vi "_iv_AUTO3.vi"(5 "i-v class":T1={"start(mV)"=0.0, "stop(mV)"=5.0, "step(mV)"=0.1, "file_name"="IV-TRx_0.00_111_test.csv", "IF OFF/ON"=TRUE, "SAVE OFF/ON"=TRUE, "frq(GHz)"=8.0, "avg"=1, "Sweep mode"=1, "VminfromSS"=0.05, "Measurement mode"=1, "Vopt"=0} {"Measurement mode" items=["Voltage sweep", "Every time HOT/COLD"]; "Sweep mode" items=["Once", "Hot/Cold auto", "HOT/Cold Manula"]}, 6 "Control":T3={"GPIB_ATT"="28", "6501Dev#"=1, "GPIB_SP"="18", "GPIB_PM"="13", "GPIB_DSA"="11", "GPIB_DMM (TPD)"="23", "GPIB_MPI"="2", "mortor setup"=[{"Axis"=0, "ID"=0, "HIspeed"=200.0, "LOspeed"=100.0, "ACCEL(ms)"=100.0, "Sratio"=50.0, "free ride"=TRUE, "string"="DSB HOT/COLD"}, {"Axis"=1, "ID"=0, "HIspeed"=4.0, "LOspeed"=4.0, "ACCEL(ms)"=100.0, "Sratio"=50.0, "free ride"=TRUE, "string"="SubMM Att"}], "DATA path"=path "Z:/band10/Labview_ALMA/MIX95/test", "DB path"=path "Z:/band10/Labview_ALMA/MIX95/test", "comment"="P1_Tmin", "ColdCarts"="003601", "Th"=295.0, "Tc"=77.0, "Set_SIS_volt"=2.1, "Offset"=0.0, "control"=0, "FreqLO"=800.0, "Set_Mag_Cur"=800.0, "MPI offset(mm)"=22.99, "HOT/COLD"=0} {"HOT/COLD" items=["DSB", "SBR", "GainComp"]; "control" items=["CLOSE LOOP", "OPEN LOOP", "Not Control"]}, 7 "Bias_LO_equip":T2={"Node address"=19, "CAN Interface"="CAN0", "Cartridge band"=10, "Slave Node in"={"Address"=0, "Serial Number"=[]}, "ObjHandle out"=0, "POL"=1, "sb"=1, "GPIB_SM (SIS S,V)"="24", "GPIB_DMM (SIS I)"="22", "GPIB_SM (MAG I) "="25", "GPIB_SG(LO)"="19", "GPIB_PW (PAMP) "="6", "GPIB_TMP1(8ch)"="12", "GPIB_TMP2(2ch)  "="13", "WCA_avg"=10, "Rsen"=10.0, "BiasModule"=1, "LOModule "=1, "WCA_LO_FREQ_SET"={"YTO Low freq. [GHz]"=14.42, "YTO High freq. [GHz]"=17.7, "Kvco"=1, "Lock Pol."=0, "SET LO FREQ"=72.5, "Multiplier"=6.0, "YTO (HEX)"=0, "YTO coarse( FREQ)"=25.0, "NULL PLL INTEGRATOR"=FALSE}, "Res for"=0} {"Res for" items=["none", "series res", "parallel res"]; "WCA_LO_FREQ_SET"."YTO coarse( FREQ)" min=25 max=150 step=0.0001 format="%.3f"; "WCA_LO_FREQ_SET"."Multiplier" min=3 max=6 step=3; "WCA_LO_FREQ_SET"."SET LO FREQ" min=25 max=150 step=0.0001 format="%.3f"; "WCA_LO_FREQ_SET"."Lock Pol." items=["Lower", "Upper"]; "WCA_LO_FREQ_SET"."Kvco" items=["7.5MHz/V", "15MHz/V"]; "WCA_LO_FREQ_SET"."YTO High freq. [GHz]" format="%.3f"; "WCA_LO_FREQ_SET"."YTO Low freq. [GHz]" format="%.3f"; "LOModule" items=["Manual", "B10Lab LO", "WCA LO"]; "BiasModule" items=["B10Lab Bias", "WCA BiasModule"]; "Slave Node in"."Serial Number" format="%.0x"; "Slave Node in"."Address" format="%.0x"; "Cartridge band" max=10 step=1; "Node address" format="%.0x"}) -> (0 "Output string":string, 1 "Set_SIS_volt":dbl=2.1, 2 "XY graph 3":cluster{dbl[], dbl[]}(graph), 3 "XY graph 2":cluster{dbl[], dbl[]}(graph))   [LabVIEW 2017]
uses:
  Instance           3 17Saved   _iv_AUTO3 .vi
  Instance           2 17Saved   _iv_AUTO3 .vi
  <vilib>/express/express shared/transition.llb/Dynamic To Waveform Array.vi
  <vilib>/express/express arith-compare/Formula/Block/exnFormulaBlock how many pts in the wave.vi
  <vilib>/express/express shared/ex_Modify Signal Name.vi
  <vilib>/express/express shared/transition.llb/Waveform Array To Dynamic.vi
  Instance           4 17Saved   _iv_AUTO3 .vi
  <vilib>/express/express arith-compare/Formula/XNode/ExpressFormulaBlockNode.xnode
panel:
  in  "Controller":enum32{"Page 1", "Page 2"}(tab)=enum."Page 2"
  out "XY graph":cluster{dbl[], dbl[]}[](graph)
  out "string":string
  in  "OK":bool
  # "LO freq. [GHz]"
  # "YTO LOW\n/High Freq."
  # "ZERO Intgrtr"
  # "Node Address"
  # "Serial Number"
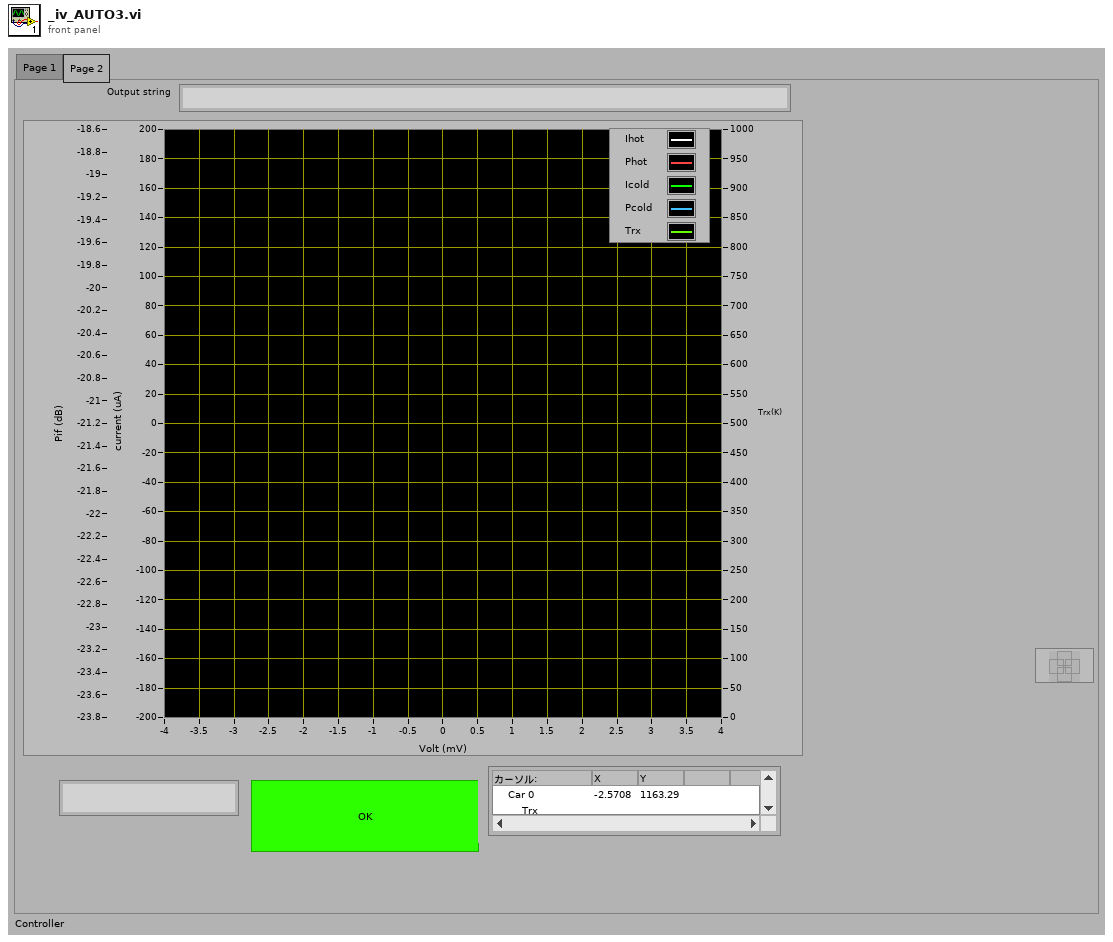
[diagram p1: front panel]
types:
  T1 = cluster{"start(mV)":dbl, "stop(mV)":dbl, "step(mV)":dbl, "file_name":string, "IF OFF/ON":bool, "SAVE OFF/ON":bool, "frq(GHz)":dbl, "avg":i32, "Sweep mode":u16, "VminfromSS":dbl, "Measurement mode":u16, "Vopt":u16}
  T2 = cluster{"Node address":u16, "CAN Interface":string, "Cartridge band":u32, "Slave Node in":cluster{"Address":i16, "Serial Number":i8[]}, "ObjHandle out":u32, "POL":u32, "sb":u32, "GPIB_SM (SIS S,V)":string, "GPIB_DMM (SIS I)":string, "GPIB_SM (MAG I) ":string, "GPIB_SG(LO)":string, "GPIB_PW (PAMP) ":string, "GPIB_TMP1(8ch)":string, "GPIB_TMP2(2ch)  ":string, "WCA_avg":i32, "Rsen":dbl, "BiasModule":u16, "LOModule ":u16, "WCA_LO_FREQ_SET":cluster{"YTO Low freq. [GHz]":sgl, "YTO High freq. [GHz]":sgl, "Kvco":u16, "Lock Pol.":u16, "SET LO FREQ":sgl, "Multiplier":sgl, "YTO (HEX)":u16, "YTO coarse( FREQ)":sgl, "NULL PLL INTEGRATOR":bool}, "Res for":u16}
  T3 = cluster{"GPIB_ATT":string, "6501Dev#":i16, "GPIB_SP":string, "GPIB_PM":string, "GPIB_DSA":string, "GPIB_DMM (TPD)":string, "GPIB_MPI":string, "mortor setup":cluster{"Axis":i16, "ID":i16, "HIspeed":dbl, "LOspeed":dbl, "ACCEL(ms)":dbl, "Sratio":dbl, "free ride":bool, "string":string}[], "DATA path":path, "DB path":path, "comment":string, "ColdCarts":string, "Th":dbl, "Tc":dbl, "Set_SIS_volt":dbl, "Offset":dbl, "control":u16, "FreqLO":dbl, "Set_Mag_Cur":dbl, "MPI offset(mm)":dbl, "HOT/COLD":u16}
  T4 = cluster{"Axis":i16, "ID":i16, "HIspeed":dbl, "LOspeed":dbl, "ACCEL(ms)":dbl, "Sratio":dbl, "free ride":bool, "string":string}[]
  T5 = cluster{"Axis":i16, "ID":i16, "HIspeed":dbl, "LOspeed":dbl, "ACCEL(ms)":dbl, "Sratio":dbl, "free ride":bool, "string":string}
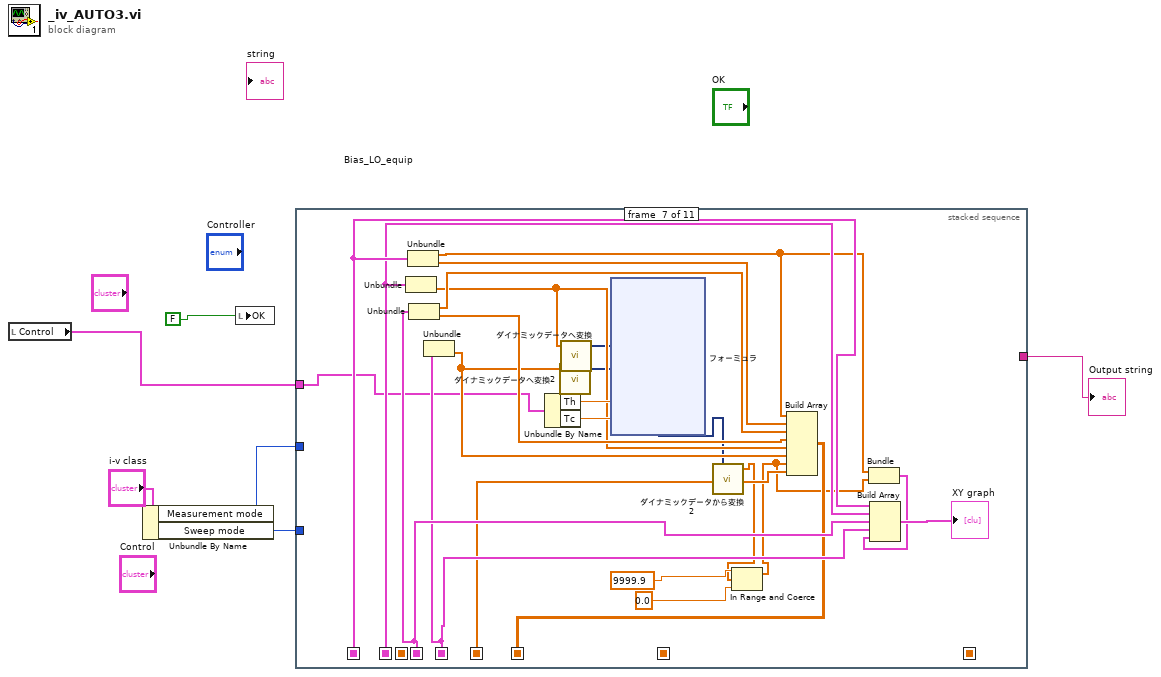
[diagram p0: block diagram]
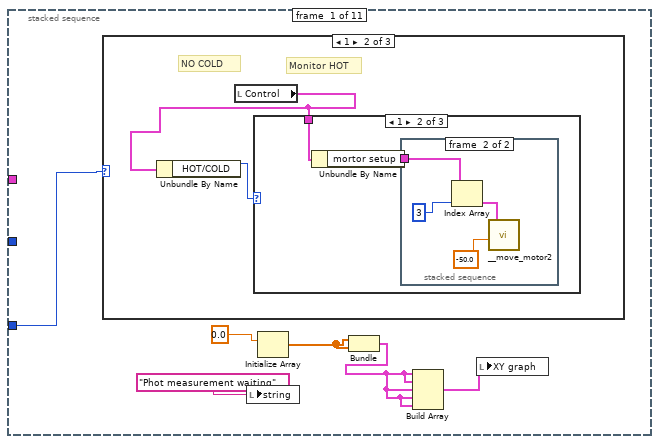
[diagram p2: hidden frame]
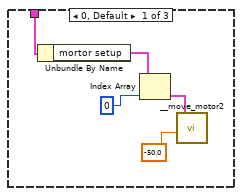
[diagram p4: hidden frame]
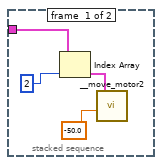
[diagram p5: hidden frame]
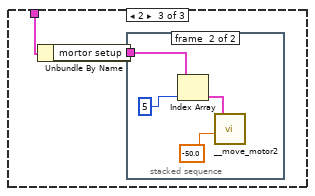
[diagram p6: hidden frame]
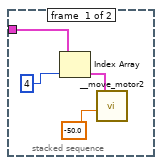
[diagram p7: hidden frame]
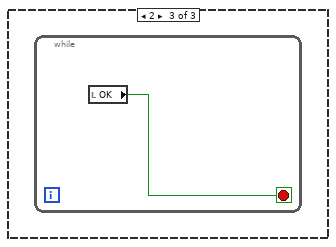
[diagram p8: hidden frame]
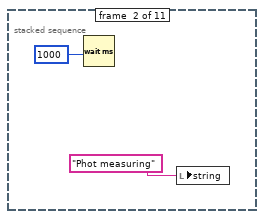
[diagram p9: hidden frame]
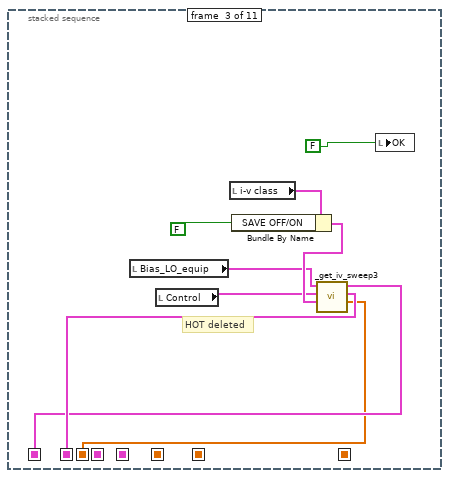
[diagram p10: hidden frame]
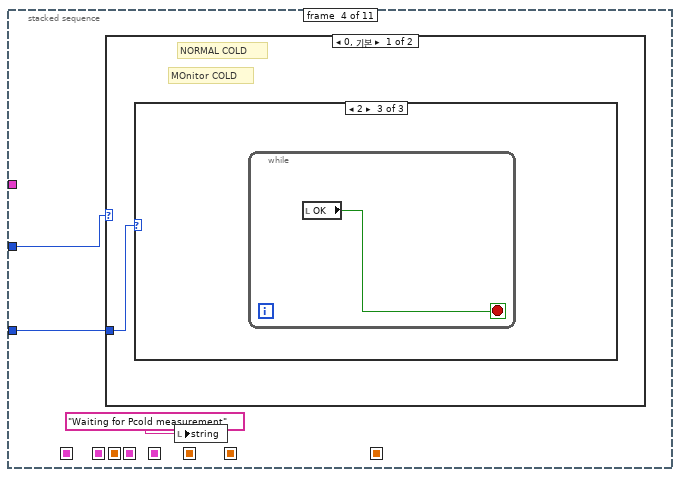
[diagram p11: hidden frame]
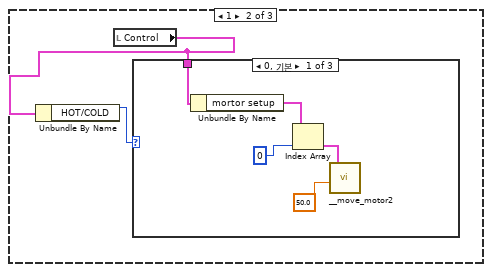
[diagram p13: hidden frame]
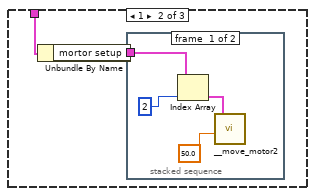
[diagram p14: hidden frame]
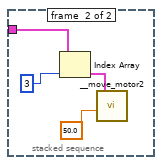
[diagram p15: hidden frame]
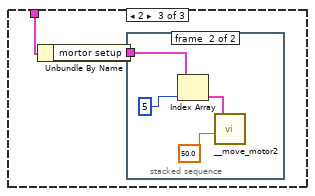
[diagram p16: hidden frame]
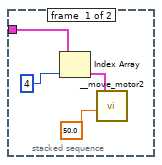
[diagram p17: hidden frame]
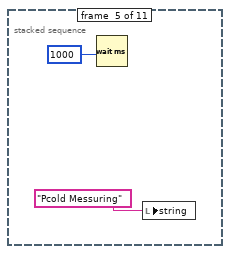
[diagram p19: hidden frame]
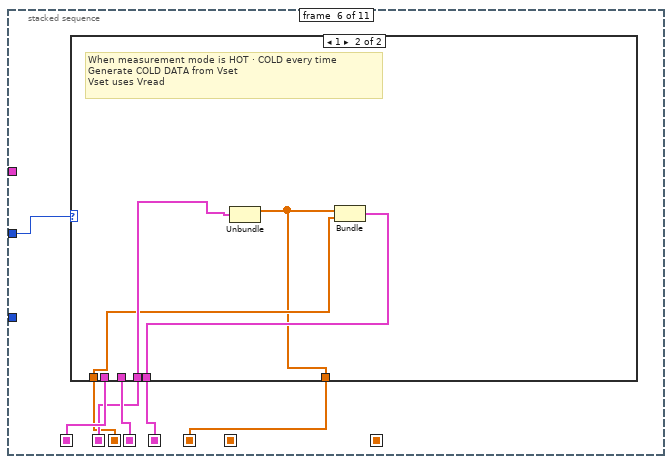
[diagram p20: hidden frame]
diagram:
  n1 = local read "Control"() -> (w5:T3)
  n2 = Unbundle By Name("i-v class") -> ("Measurement mode"=w3:u16, "Sweep mode"=w2:u16)
  n3 = local write "OK"(FALSE) -> ()
  n4 = stacked-sequence {
    seq-local: [_ _ w45 _ _ _ _ _ _ _ _] -> [_ _ _ _ _ w88 w125 _ _ _ _]
    seq-local: [_ _ w50 _ _ _ _ _ _ _ _] -> [_ _ _ _ _ w87 w124 _ _ _ _]
    seq-local: [_ _ _ _ _ w91 _ _ _ _ _] -> [_ _ _ _ _ _ w123 _ _ _ _]
    seq-local: [_ _ _ _ _ w90 _ _ _ _ _] -> [_ _ _ _ _ _ w122 _ _ _ _]
    seq-local: [_ _ _ _ _ w92 _ _ _ _ _] -> [_ _ _ _ _ _ w112 _ _ _ _]
    seq-local: [_ _ _ _ _ _ w110 _ _ _ _] -> [_ _ _ _ _ _ _ w271 w289 _ _]
    seq-local: [_ _ _ _ _ _ _ _ w290 _ _] -> [_ _ _ _ _ _ _ _ _ w356 _]
    seq-local: [_ _ _ _ _ _ _ _ _ w339 _] -> [_ _ _ _ _ _ _ _ _ _ w372]
    seq-local: [_ _ w44 _ _ _ _ _ _ _ _] -> [_ _ _ _ _ w86 _ _ _ _ _]
    tunnel: w5 -> [_ _ _ _ _ _ w109 w268 _ _ _]
    tunnel: [_ _ _ _ _ _ _ _ _ w338 _] -> w6
    tunnel: w3 -> [_ _ _ w54 _ w89 _ _ _ _ _]
    tunnel: w2 -> [w8 _ _ w53 _ _ _ _ _ _ _]
    frame #0 {
      n5 = case shown="1" w8 {
        frame 0, Default {
        }
        frame 1 {
          # "NO COLD"
          # "Monitor HOT"
          n6 = local read "Control"() -> (w13:T3)
          n7 = Unbundle By Name(w13) -> ("HOT/COLD"=w14:u16)
          n8 = case shown="1" w14 {
            tunnel: w13 -> [w17 w21 w31]
            frame 0, Default {
              n9 = Unbundle By Name(w17) -> ("mortor setup"=w16:T4)
              n10 = Index Array(array=w16, index=0) -> (element=w15:T5)
              n11 = call "__move_motor2.vi"("Moving distance"=-50.0, "motor setup"=w15) -> ()  [unwired: 2 in, 2 out]
            }
            frame 1 {
              n12 = Unbundle By Name(w21) -> ("mortor setup"=w20:T4)
              n13 = stacked-sequence {
                tunnel: w20 -> [w23 w27]
                frame #0 {
                  n14 = Index Array(array=w23, index=2) -> (element=w22:T5)
                  n15 = call "__move_motor2.vi"("Moving distance"=-50.0, "motor setup"=w22) -> ()  [unwired: 2 in, 2 out]
                }
                frame #1 {
                  n16 = Index Array(array=w27, index=3) -> (element=w26:T5)
                  n17 = call "__move_motor2.vi"("Moving distance"=-50.0, "motor setup"=w26) -> ()  [unwired: 2 in, 2 out]
                }
              }
            }
            frame 2 {
              n18 = Unbundle By Name(w31) -> ("mortor setup"=w30:T4)
              n19 = stacked-sequence {
                tunnel: w30 -> [w33 w37]
                frame #0 {
                  n20 = Index Array(array=w33, index=4) -> (element=w32:T5)
                  n21 = call "__move_motor2.vi"("Moving distance"=-50.0, "motor setup"=w32) -> ()  [unwired: 2 in, 2 out]
                }
                frame #1 {
                  n22 = Index Array(array=w37, index=5) -> (element=w36:T5)
                  n23 = call "__move_motor2.vi"("Moving distance"=-50.0, "motor setup"=w36) -> ()  [unwired: 2 in, 2 out]
                }
              }
            }
          }
        }
        frame 2 {
          n24 = while {
            stop <- w40 stop-if-true
            n25 = local read "OK"() -> (w40:bool)
          }
        }
      }
      n26 = local write "string"("Phot measurement waiting") -> ()
      n27 = Initialize Array(0.0) -> (w12:dbl[])  [unwired: 1 in]
      n28 = Bundle(w12, w12) -> (w9:cluster{dbl[], dbl[]})  [unwired: 1 in]
      n29 = Build Array(w9, w9, w9, w9, w9) -> (w10:cluster{dbl[], dbl[]}[])
      n30 = local write "XY graph"(w10) -> ()
    }
    frame #1 {
      n31 = Wait (ms)(milliseconds to wait=1000) -> ()  [unwired: 1 out]
      n32 = local write "string"("Phot measuring") -> ()
    }
    frame #2 {
      # "HOT deleted"
      n33 = local read "Bias_LO_equip"() -> (w47:T2)
      n34 = local read "Control"() -> (w46:T3)
      n35 = local read "i-v class"() -> (w49:T1)
      n36 = Bundle By Name(cluster=w49, "SAVE OFF/ON"=FALSE) -> (w48:T1)
      n37 = call "_get_iv_sweep3.vi"("I-V class"=w48, "Control"=w46, "Bias_LO_equip"=w47) -> ("Vset"=w44:dbl[], "VP class"=w50:cluster{"array":dbl[], "array2":dbl[]}, "VI class"=w45:cluster{"array":dbl[], "array2":dbl[]})  [unwired: 2 in]
      n38 = local write "OK"(FALSE) -> ()
    }
    frame #3 {
      n39 = case shown="0, 기본" w54 {
        tunnel: w53 -> [w55 _]
        frame 0, Default {
          # "NORMAL COLD"
          # "MOnitor COLD"
          n40 = case shown="2" w55 {
            frame 0, Default {
            }
            frame 1 {
              n41 = local read "Control"() -> (w56:T3)
              n42 = Unbundle By Name(w56) -> ("HOT/COLD"=w57:u16)
              n43 = case shown="0, 기본" w57 {
                tunnel: w56 -> [w60 w64 w74]
                frame 0, Default {
                  n44 = Unbundle By Name(w60) -> ("mortor setup"=w59:T4)
                  n45 = Index Array(array=w59, index=0) -> (element=w58:T5)
                  n46 = call "__move_motor2.vi"("Moving distance"=50.0, "motor setup"=w58) -> ()  [unwired: 2 in, 2 out]
                }
                frame 1 {
                  n47 = Unbundle By Name(w64) -> ("mortor setup"=w63:T4)
                  n48 = stacked-sequence {
                    tunnel: w63 -> [w66 w70]
                    frame #0 {
                      n49 = Index Array(array=w66, index=2) -> (element=w65:T5)
                      n50 = call "__move_motor2.vi"("Moving distance"=50.0, "motor setup"=w65) -> ()  [unwired: 2 in, 2 out]
                    }
                    frame #1 {
                      n51 = Index Array(array=w70, index=3) -> (element=w69:T5)
                      n52 = call "__move_motor2.vi"("Moving distance"=50.0, "motor setup"=w69) -> ()  [unwired: 2 in, 2 out]
                    }
                  }
                }
                frame 2 {
                  n53 = Unbundle By Name(w74) -> ("mortor setup"=w73:T4)
                  n54 = stacked-sequence {
                    tunnel: w73 -> [w77 w80]
                    frame #0 {
                      n55 = Index Array(array=w77, index=4) -> (element=w76:T5)
                      n56 = call "__move_motor2.vi"("Moving distance"=50.0, "motor setup"=w76) -> ()  [unwired: 2 in, 2 out]
                    }
                    frame #1 {
                      n57 = Index Array(array=w80, index=5) -> (element=w79:T5)
                      n58 = call "__move_motor2.vi"("Moving distance"=50.0, "motor setup"=w79) -> ()  [unwired: 2 in, 2 out]
                    }
                  }
                }
              }
            }
            frame 2 {
              n59 = while {
                stop <- w83 stop-if-true
                n60 = local read "OK"() -> (w83:bool)
              }
            }
          }
        }
        frame 1 {
          # "When the measurement mode is HOT / COLD every time, do nothing"
        }
      }
      n61 = local write "string"("Waiting for Pcold measurement") -> ()
    }
    frame #4 {
      n62 = Wait (ms)(milliseconds to wait=1000) -> ()  [unwired: 1 out]
      n63 = local write "string"("Pcold Messuring") -> ()
    }
    frame #5 {
      n64 = case shown="1" w89 {
        tunnel: [w96 w100] -> w92
        tunnel: [w94 w104] -> w91
        tunnel: [w93 w101] -> w90
        tunnel: w88 -> [_ w104]
        tunnel: w87 -> [_ w103]
        tunnel: w86 -> [_ w102]
        frame 0, Default {
          # "COLD data acquisition"
          n65 = local read "Bias_LO_equip"() -> (w95:T2)
          n66 = local read "i-v class"() -> (w98:T1)
          n67 = Bundle By Name(cluster=w98, "SAVE OFF/ON"=FALSE) -> (w97:T1)
          n68 = call "_get_iv_sweep3.vi"("I-V class"=w97, "Bias_LO_equip"=w95) -> ("Vset"=w96:dbl[], "VP class"=w93:cluster{"array":dbl[], "array2":dbl[]}, "VI class"=w94:cluster{"array":dbl[], "array2":dbl[]})  [unwired: 3 in]
          "XY graph 2" <- w94
          "XY graph 3" <- w93
        }
        frame 1 {
          # "When measurement mode is HOT · COLD every time\nGenerate COLD DATA from Vset\nVset uses Vread"
          n69 = Unbundle(w103) -> ("array"=w100:dbl[])  [unwired: 1 out]
          n70 = Bundle("array"=w100, "Vset"=w102) -> (w101:cluster{"array":dbl[], "Vset":dbl[]})  [unwired: 1 in]
        }
      }
    }
    frame #6 {
      n71 = Unbundle(w124) -> ("array2"=w117:dbl[])  [unwired: 1 out]
      n72 = Unbundle(w125) -> ("array"=w121:dbl[], "array2"=w127:dbl[])
      n73 = Unbundle(w123) -> ("array"=w126:dbl[], "array2"=w128:dbl[])
      n74 = Unbundle(w122) -> ("Vset"=w115:dbl[])  [unwired: 1 out]
      n75 = Unbundle By Name(w109) -> ("Th"=w119:dbl, "Tc"=w118:dbl)
      n76 = call "ダイナミックデータへ変換2"("Array"=w115) -> ("Dynamic Data Type"=w114:dynamicdata)  [unwired: 3 in]
      n77 = call "ダイナミックデータへ変換"("Array"=w117) -> ("Dynamic Data Type"=w116:dynamicdata)  [unwired: 3 in]
      n78 = xnode "フォーミュラ"("Ph"=w116, "Pc"=w114, "th"=w119, "tc"=w118) -> ("결과"=w113:dynamicdata)  [unwired: 1 in, 1 out]
      n79 = call "ダイナミックデータから変換2"("Dynamic Data Type"=w113) -> ("Array"=w106:dbl[])  [unwired: 3 in]
      n80 = In Range and Coerce(upper limit=9999.9, x=w106, lower limit=0.0) -> (coerced(x)=w105:dbl[])  [unwired: 1 out]
      n81 = Build Array(w121, w127, w126, w128, w117, w115, w105, w112) -> (w110:dbl[][])
      n82 = Bundle("array"=w121, w105) -> (w111:cluster{"array":dbl[], dbl[]})  [unwired: 1 in]
      n83 = Build Array(w125, w124, w123, w122, w111) -> (→"XY graph":cluster{"array":dbl[], "Vset":dbl[]}[])
    }
    frame #7 {
      n84 = local read "i-v class"() -> (w269:T1)
      n85 = Unbundle By Name(w269) -> ("SAVE OFF/ON"=w270:bool)
      n86 = case shown="참" w270 {
        tunnel: w271 -> [_ w278]
        tunnel: w269 -> [_ w276]
        tunnel: w268 -> [_ w274]
        frame False {
        }
        frame True {
          n87 = Unbundle By Name(w276) -> ("file_name"=w275:string)
          n88 = Unbundle By Name(w274) -> ("DATA path"=w273:path, "Offset"=w272:dbl)
          n89 = Format Into String(format string="Vsis,Ihot,Vcold,Icold,Phot,Pcold,Trx,Vset with Offset=%f", w272) -> (resulting string=w279:string)  [unwired: 2 in, 1 out]
          n90 = call "___save_2d_data_with_header.vi"("ヘッダー"=w279, "”z—ñ"=w278, "Œ`Ž®"="%^.3e", "file_name"=w275, "パス"=w273) -> ()  [unwired: 6 in, 1 out]
        }
      }
    }
    frame #8 {
      n91 = local read "i-v class"() -> (w285:T1)
      n92 = local read "Control"() -> (w287:T3)
      n93 = Unbundle By Name(w285) -> ("Vopt"=w281:u16, "VminfromSS"=w283:dbl)
      n94 = Array Size(array=w289) -> (size(s)=w293:i32[])
      n95 = Index Array(array=w293, index=1) -> (element=w291:i32)
      n96 = Unbundle By Name(w287) -> ("FreqLO"=w286:dbl)
      n97 = expression code="2.0678E -3*x"(w286) -> (w284:dbl)
      n98 = Add(x=w284, y=w283) -> (x+y=w282:dbl)
      n99 = case shown="1" w281 {
        tunnel: w291 -> [_ w299 w319]
        tunnel: [w294 w298 w318] -> w290
        tunnel: w289 -> [w294 w297 w317]
        tunnel: dbl[][] [] -> [_ w296 w316]
        tunnel: w282 -> [_ w295 w315]
        frame 0, Default {
        }
        frame 1 {
          n100 = for {
            N: w299 -> [_]
            tunnel: w297 -> [w306]
            shift-right: [w305] -> w298
            shift-left: w296 -> [w304]
            tunnel: w295 -> [w300]
            i -> [w302]
            n101 = Index Array(array=w306, index (row)=0, index (col)=w302) -> (element=w308:dbl)
            n102 = In Range and Coerce(upper limit=2.3, x=w308, lower limit=w300) -> (In Range?=w307:bool)  [unwired: 1 out]
            n103 = case shown="참" w307 {
              tunnel: w302 -> [_ w310]
              tunnel: w306 -> [_ w314]
              tunnel: [w309 w312] -> w305
              tunnel: w304 -> [w309 w311]
              frame False {
              }
              frame True {
                n104 = Index Array(array=w314, index (col)=w310) -> (element=w313:dbl[])  [unwired: 1 in]
                n105 = Build Array (concatenate)(w311, w313) -> (w312:dbl[][])
              }
            }
          }
        }
        frame 2 {
          n106 = for {
            N: w319 -> [_]
            tunnel: w317 -> [w327]
            shift-right: [w326] -> w318
            shift-left: w316 -> [w325]
            tunnel: w315 -> [w320]
            i -> [w323]
            n107 = Index Array(array=w327, index (row)=0, index (col)=w323) -> (element=w329:dbl)
            n108 = Negate(x=w320) -> (-x=w321:dbl)
            n109 = In Range and Coerce(upper limit=w321, x=w329, lower limit=-2.3) -> (In Range?=w328:bool)  [unwired: 1 out]
            n110 = case shown="참" w328 {
              tunnel: w323 -> [_ w331]
              tunnel: w327 -> [_ w335]
              tunnel: [w330 w333] -> w326
              tunnel: w325 -> [w330 w332]
              frame False {
              }
              frame True {
                n111 = Index Array(array=w335, index (col)=w331) -> (element=w334:dbl[])  [unwired: 1 in]
                n112 = Build Array (concatenate)(w332, w334) -> (w333:dbl[][])
              }
            }
          }
        }
      }
    }
    frame #9 {
      n113 = Index Array(array=w356, index (col)=6) -> (element=w358:dbl[])  [unwired: 1 in]
      n114 = Array Size(array=w358) -> (size(s)=w357:i32)
      n115 = for {
        N: w357 -> [_]
        tunnel: w358 -> [w367]
        tunnel: [w363] -> w359 mode=indexing
        i -> [w368]
        n116 = Index Array(array=w367, index=w368) -> (element=w362:dbl)
        n117 = In Range and Coerce(upper limit=9999.9, x=w362, lower limit=80.0) -> (In Range?=w364:bool)  [unwired: 1 out]
        n118 = case shown="참" w364 {
          tunnel: [9999.9 w370] -> w363
          tunnel: w362 -> [_ w370]
          frame False {
          }
          frame True {
          }
        }
      }
      n119 = Array Max & Min(array=w359) -> (min index (indices)=w360:i32)  [unwired: 3 out]
      n120 = Index Array(array=w356, index (row)=w360) -> (element=w361:dbl[])  [unwired: 1 in]
      n121 = Get Date/Time In Seconds() -> (seconds since 1Jan1904=w354:timestamp)
      n122 = Format Date/Time String(time format string (%c)="%Y-%m-%d  %H:%M:%S", seconds (now)=w354) -> (date/time string=w344:string)  [unwired: 1 in]
      n123 = local read "Control"() -> (w337:T3)
      n124 = local read "Bias_LO_equip"() -> (w355:T2)
      n125 = formula code="float32 VJ,IJ;\nfloat32 Vset,Trx,Ph,Pc;\nVJ=ar[0];\nIJ=ar[1];\nVset=ar[7];\nPh=ar[4];\nPc=ar[5];\nTrx=ar[6];"("ar"=w361) -> ("VJ"=w347:sgl, "IJ"=w346:sgl, "Trx"=w348:sgl, "Vset"=w339:sgl, "Ph"=w350:sgl, "Pc"=w349:sgl)
      n126 = Unbundle By Name(w337) -> ("FreqLO"=w351:dbl)
      n127 = Unbundle By Name(w337) -> ("comment"=w340:string)
      n128 = Unbundle By Name(w355) -> ("BiasModule"=w343:u16, "LOModule"=w342:u16, "POL"=w341:u32)
      n129 = Unbundle By Name(w337) -> ("Offset"=w345:dbl)
      n130 = Format Into String(format string="IVTrx,%.2f,%2.2f,%2.2f,%.1f,%2.2f,%4.1f,%2.2f,%.3f,%s,%d,%d,%d,%s", w351, w350, w349, w348, w347, w346, w339, w345, w344, w343, w342, w341, w340) -> (resulting string=w338:string)  [unwired: 2 in, 1 out]
    }
    frame #10 {
      n131 = local read "i-v class"() -> (w375:T1)
      n132 = Unbundle By Name(w375) -> ("Vopt"=w374:u16)
      n133 = case shown="0, 기본" w374 {
        tunnel: w372 -> [w376 _]
        tunnel: [w376 w381] -> w371
        frame 1, 2 {
          n134 = local read "Control"() -> (w377:T3)
          n135 = local read "Bias_LO_equip"() -> (w378:T2)
          n136 = Unbundle By Name(w377) -> ("Offset"=w380:dbl, "control"=w379:u16)
          n137 = call "__SISbias_Set.vi"("SIS@Mode"=w379, "Offset"=w380, "Set_V"=w376, "Bias_LO_equip"=w378) -> ()  [unwired: 7 in, 1 out]
        }
        frame 0, Default {
          n138 = local read "Control"() -> (w382:T3)
          n139 = local read "Bias_LO_equip"() -> (w383:T2)
          n140 = Unbundle By Name(w382) -> ("Offset"=w385:dbl, "control"=w384:u16, "Set_SIS_volt"=w381:dbl)
          n141 = call "__SISbias_Set.vi"("SIS@Mode"=w384, "Offset"=w385, "Set_V"=w381, "Bias_LO_equip"=w383) -> ()  [unwired: 7 in, 1 out]
        }
      }
      "Set_SIS_volt" <- w371
      n142 = local write "string"("Measurement End") -> ()
    }
  }
  "Output string" <- w6
